vi "2D Gaussian Smooth.vi"(9 "radius":u16=2, 11 "Input":dbl[][](graph)) -> (0 "Margin":u16=6, 3 "Output":dbl[][](graph))   [LabVIEW 2018]
uses:
  <vilib>/Analysis/2dsp.llb/1D Convolution (DBL).vi
  <vilib>/Analysis/NI_AALPro.lvlib
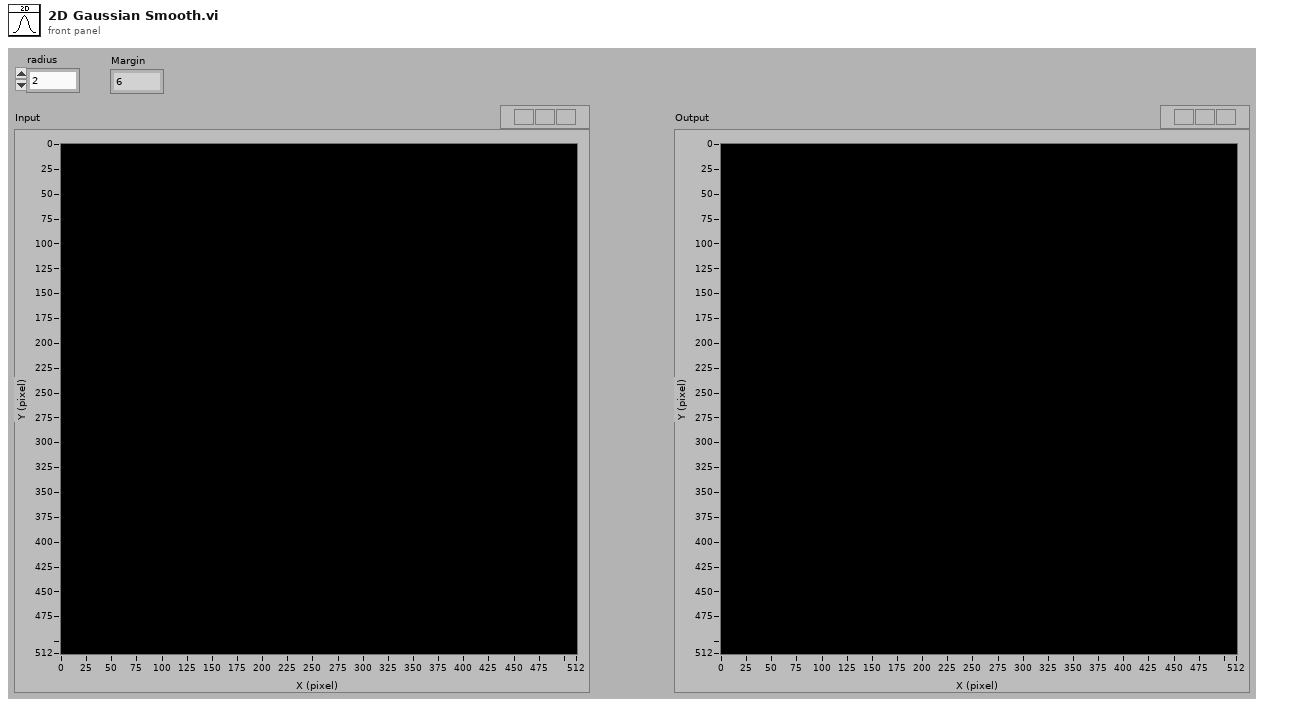
[diagram p1: front panel]
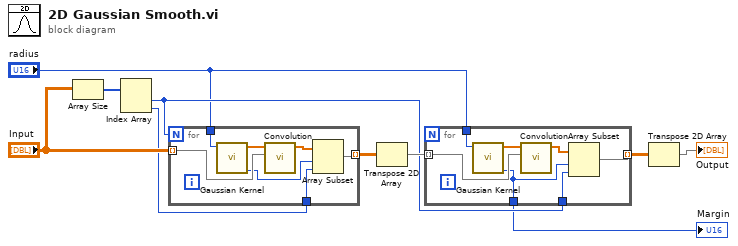
[diagram p0: block diagram]
diagram:
  n1 = Array Size(array="Input") -> (size(s)=w10:i32[])
  n2 = Index Array(array=w10) -> (element #1=w4:i32, element #2=w5:i32)  [unwired: 2 in]
  n3 = for {
    N: w4 -> [_]
    tunnel: "Input" -> [w14] mode=indexing
    tunnel: [w17] -> w9 mode=indexing
    tunnel: w5 -> [w16]
    tunnel: "radius" -> [w12]
    n4 = call "Gaussian Kernel.vi"("radius"=w12) -> ("1/2 Kernel size"=w11:u16, "Kernel"=w15:dbl[])  [unwired: 9 in]
    n5 = call-poly <vilib>:"Convolution.vi"("Y"=w14, "X"=w15) -> ("X * Y"=w13:dbl[])  [unwired: 8 in, 1 out]
    n6 = Array Subset(array=w13, index=w11, length=w16) -> (w17:dbl[])
  }
  n7 = Transpose 2D Array(2D array=w9) -> (transposed array=w8:dbl[][])
  n8 = for {
    tunnel: w8 -> [w20] mode=indexing
    tunnel: [w24] -> w7 mode=indexing
    tunnel: w4 -> [w23]
    tunnel: "radius" -> [w21]
    tunnel: [w18] -> w1
    n9 = call "Gaussian Kernel.vi"("radius"=w21) -> ("1/2 Kernel size"=w18:u16, "Kernel"=w22:dbl[])  [unwired: 9 in]
    n10 = call-poly <vilib>:"Convolution.vi"("Y"=w20, "X"=w22) -> ("X * Y"=w19:dbl[])  [unwired: 8 in, 1 out]
    n11 = Array Subset(array=w19, index=w18, length=w23) -> (w24:dbl[])
  }
  "Margin" <- w1
  n12 = Transpose 2D Array(2D array=w7) -> (transposed array=→"Output":dbl[][])
